vi "input_control.vi"() -> ()   [LabVIEW 2023]
panel:
  in  "stop":bool
  out "Numeric 2":dbl
  out "Numeric":dbl
  in  "String":string
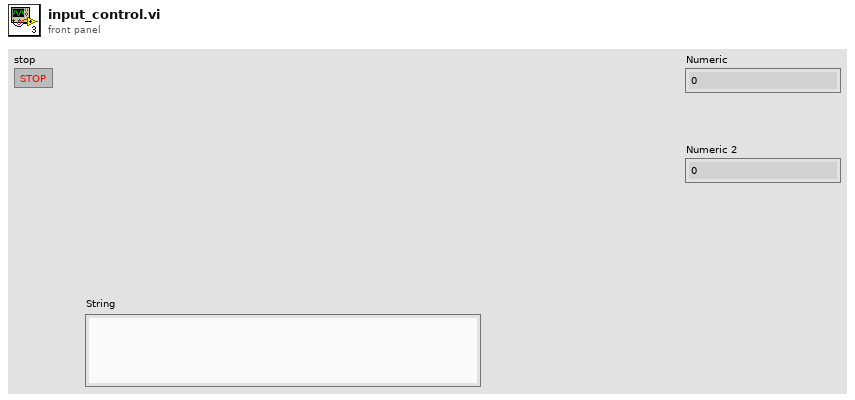
[diagram p1: front panel]
types:
  T1 = enum16{"Native", "Native Command Line", "UNIX", "Macintosh", "DOS"}
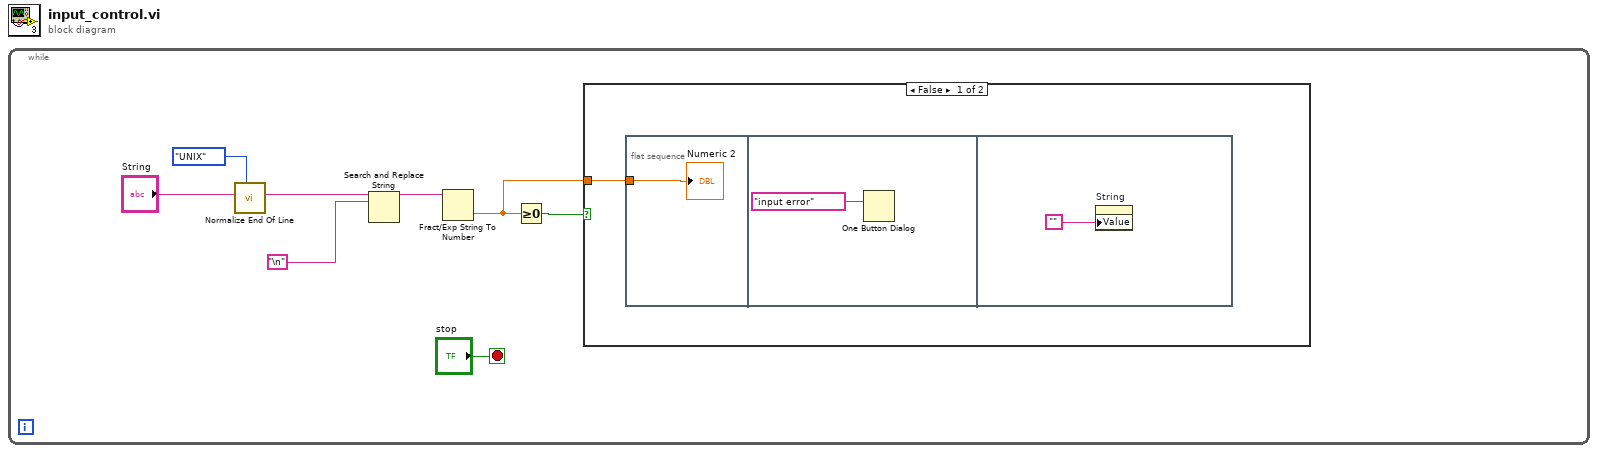
[diagram p0: block diagram]
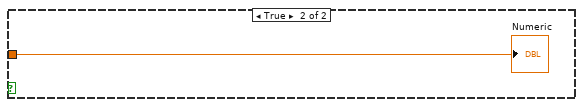
[diagram p2: hidden frame]
diagram:
  n1 = while {
    stop <- "stop" stop-if-true
    n2 = call <vilib>:"Normalize End Of Line.vi"("end of line (Native)"=T1."UNIX", "string in"="String") -> ("string out"=w2:string)  [unwired: 6 in]
    n3 = Search and Replace String(input string=w2, search string="\n") -> (result string=w7:string)  [unwired: 6 in, 3 out]
    n4 = Fract/Exp String To Number(string=w7) -> (number=w6:dbl)  [unwired: 3 in, 1 out]
    n5 = Greater Or Equal To 0?(x=w6) -> (x >= 0?=w8:bool)
    n6 = case shown="False" w8 {
      tunnel: w6 -> [w9 w13]
      frame False {
        n7 = flat-sequence {
          tunnel: w9 -> [w10]
          frame #0 {
            "Numeric 2" <- w10
          }
          frame #1 {
            n8 = One Button Dialog(message="input error") -> ()  [unwired: 1 in, 1 out]
          }
          frame #2 {
            n9 = property on="String" class="Str"("Value"="") -> ()  [unwired: 2 in, 2 out]
          }
        }
      }
      frame True {
        "Numeric" <- w13
      }
    }
  }
